vi "Slider Position Chasing.vi"(8 "Position Compensate":cluster{"Array 2":dbl[]}[](array[cluster]) {"Array 2" format="%#_f"}, 10 "Chasing Group":cluster{"Array 2":refnum<vi>[]}[](array[cluster]), 11 "Slide Reference In":refnum<vi>) -> (3 "Slide Reference Out":refnum<vi>)   [LabVIEW 2019]
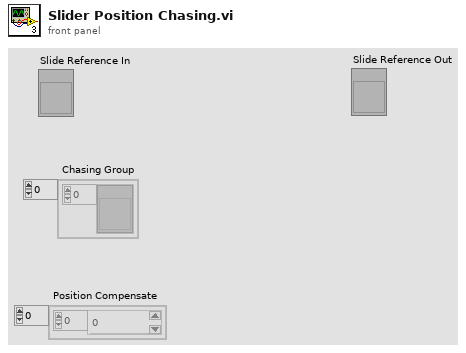
[diagram p1: front panel]
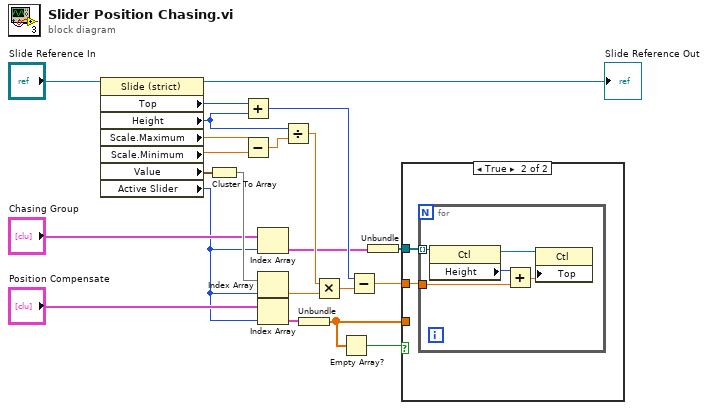
[diagram p0: block diagram]
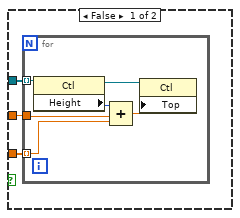
[diagram p2: hidden frame]
diagram:
  n1 = property class="Slide (strict)"(reference="Slide Reference In") -> (reference out=→"Slide Reference Out":refnum<vi>, "Top"=w21:i32, "Height"=w20:u32, "Scale.Maximum"=w19:dbl, "Scale.Minimum"=w18:dbl, "Value"=w12:cluster{dbl, dbl, dbl}, "Active Slider"=w5:i32)  [unwired: 1 in, 1 out]
  n2 = Cluster To Array(cluster=w12) -> (array=w11:dbl[])
  n3 = Add(x=w21, y=w20) -> (x+y=w15:u32)
  n4 = Subtract(x=w19, y=w18) -> (x-y=w22:dbl)
  n5 = Index Array(array="Chasing Group", index=w5) -> (element=w8:cluster{"Array 2":refnum<vi>[]})
  n6 = Index Array(array=w11, index=w5) -> (element=w10:dbl)
  n7 = Index Array(array="Position Compensate", index=w5) -> (element=w4:cluster{"Array 2":dbl[]})
  n8 = Divide(x=w20, y=w22) -> (x/y=w16:dbl)
  n9 = Unbundle(w4) -> ("Array 2"=w2:dbl[])
  n10 = Multiply(x=w16, y=w10) -> (x*y=w17:dbl)
  n11 = Empty Array?(array=w2) -> (empty?=w3:bool)
  n12 = Subtract(x=w15, y=w17) -> (x-y=w14:dbl)
  n13 = Unbundle(w8) -> ("Array 2"=w7:refnum<vi>[])
  n14 = case shown="True" w3 {
    tunnel: w14 -> [w25 w32]
    tunnel: w7 -> [w24 w33]
    tunnel: w2 -> [w23 _]
    frame False {
      n15 = for {
        tunnel: w25 -> [w27]
        tunnel: w24 -> [w28] mode=indexing
        tunnel: w23 -> [w26] mode=indexing
        n16 = property class="Ctl"(reference=w28) -> (reference out=w30:refnum<vi>, "Height"=w29:u32)  [unwired: 1 in, 1 out]
        n17 = Compound Arithmetic op=ADD(w29, w27, w26) -> (w31:dbl)
        n18 = property class="Ctl"(reference=w30, "Top"=w31) -> ()  [unwired: 1 in, 2 out]
      }
    }
    frame True {
      n19 = for {
        tunnel: w32 -> [w36]
        tunnel: w33 -> [w37] mode=indexing
        n20 = property class="Ctl"(reference=w37) -> (reference out=w38:refnum<vi>, "Height"=w35:u32)  [unwired: 1 in, 1 out]
        n21 = Add(x=w35, y=w36) -> (x+y=w34:dbl)
        n22 = property class="Ctl"(reference=w38, "Top"=w34) -> ()  [unwired: 1 in, 2 out]
      }
    }
  }
